vi "BRig_dataMtrig_init__resetCounters.vi"(11 "input_dataMTrig":u16[](array[numeric])) -> (3 "output_dataMTrig":u16[](array[numeric]))   [LabVIEW 2014]
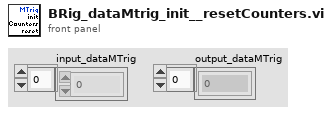
[diagram p1: front panel]
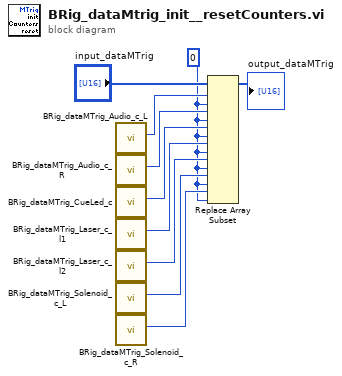
[diagram p0: block diagram]
diagram:
  w1 = u16 0 ("new element/subarray")
  n1 = call "BRig_dataMTrig_Audio_c_L.vi"() -> ("output_Audio_c_L"=w8:i32)  [unwired: 11 in]
  n2 = call "BRig_dataMTrig_Audio_c_R.vi"() -> ("output_Audio_c_R"=w7:i32)  [unwired: 11 in]
  n3 = call "BRig_dataMTrig_CueLed_c.vi"() -> ("output_CueLed_c"=w6:i32)  [unwired: 11 in]
  n4 = call "BRig_dataMTrig_Laser_c_l1.vi"() -> ("output_Laser_c_l1"=w5:i32)  [unwired: 11 in]
  n5 = call "BRig_dataMTrig_Laser_c_l2.vi"() -> ("output_Laser_c_l2"=w4:i32)  [unwired: 11 in]
  n6 = call "BRig_dataMTrig_Solenoid_c_L.vi"() -> ("output_Solenoid_c_L"=w3:i32)  [unwired: 11 in]
  n7 = call "BRig_dataMTrig_Solenoid_c_R.vi"() -> ("output_Solenoid_c_R"=w2:i32)  [unwired: 11 in]
  n8 = Replace Array Subset(array="input_dataMTrig", new element #1=w1, index #1=w8, new element #2=w1, index #2=w7, new element #3=w1, index #3=w6, new element #4=w1, index #4=w5, new element #5=w1, index #5=w4, new element #6=w1, index #6=w3, new element #7=w1, index #7=w2) -> (→"output_dataMTrig":u16[])
